vi "ForceSensor_Final.vi"() -> ()   [LabVIEW 2020]
uses:
  <vilib>/Analysis/baseanly.llb/Mean (DBL).vi
  <vilib>/httpClient/PUTBuffer.vi
  <vilib>/httpClient/LabVIEWHTTPClient.lvlib
  <vilib>/ptbypt/NI_PtbyPt.lvlib
  <vilib>/Analysis/NI_AALBase.lvlib
panel:
  out "Waveform Chart 2":dynamicdata(graph)
  out "Cloud payload":string
  out "Waveform Chart":dynamicdata(graph)
  out "x > y?":bool
  in  "Calibration Tap":bool
  in  "Calibration Reset":bool
  out "BPM":dbl
  in  "stop":bool
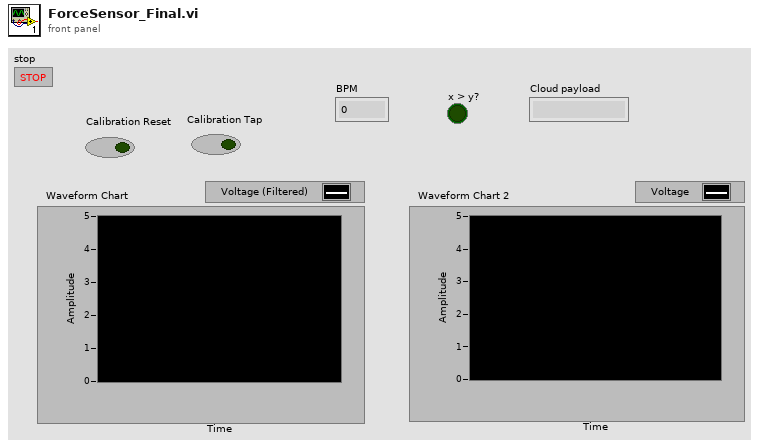
[diagram p1: front panel]
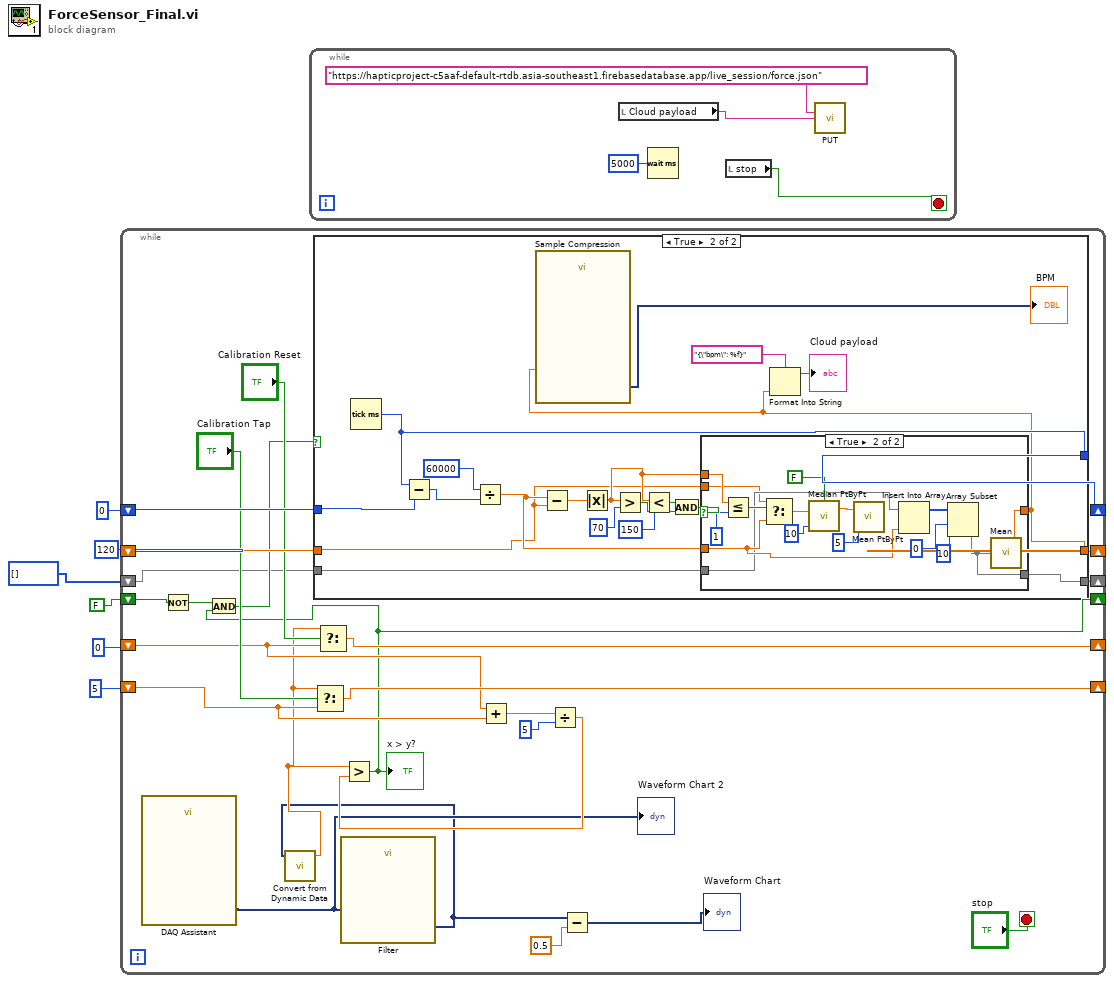
[diagram p0: block diagram]
diagram:
  n1 = while {
    shift-right: [w29] -> _
    shift-left: 0 -> [w30]
    shift-right: [w27] -> _
    shift-left: 120 -> [w28]
    shift-right: [w24] -> _
    shift-left: 0 -> [w22]
    shift-right: [w23] -> _
    shift-left: 5 -> [w21]
    shift-right: [w13] -> _
    shift-left: FALSE -> [w16]
    shift-right: [w11] -> _
    shift-left: i32[] [] -> [w12]
    stop <- "stop" stop-if-true
    n2 = call "DAQ Assistant"() -> ("data"=w10:dynamicdata)  [unwired: 16 in, 3 out]
    "Waveform Chart 2" <- w10
    n3 = Not(x=w16) -> (.not. x?=w15:bool)
    n4 = call "Filter"("Signal"=w10) -> ("Filtered Signal"=w9:dynamicdata)  [unwired: 9 in, 1 out]
    n5 = call "Convert from Dynamic Data"("Dynamic Data Type"=w9) -> ("Scalar"=w17:dbl)  [unwired: 3 in]
    n6 = Select(t=w17, s="Calibration Tap", f=w21) -> (s? t:f=w23:dbl)
    n7 = Select(t=w17, s="Calibration Reset", f=w22) -> (s? t:f=w24:dbl)
    n8 = Add(x=w22, y=w21) -> (x+y=w20:dbl)
    n9 = Divide(x=w20, y=5) -> (x/y=w18:dbl)
    n10 = Greater?(x=w17, y=w18) -> (0:w13:bool)
    "x > y?" <- w13
    n11 = And(x=w15, y=w13) -> (x .and. y?=w14:bool)
    n12 = case shown="True" w14 {
      tunnel: w30 -> [w34 w53]
      tunnel: [w34 w50] -> w29
      tunnel: w28 -> [w33 w37]
      tunnel: [w33 w35] -> w27
      tunnel: w12 -> [w32 w39]
      tunnel: [w32 w38] -> w11
      frame False {
      }
      frame True {
        n13 = Tick Count (ms)() -> (millisecond timer value=w50:u32)
        n14 = Subtract(x=w50, y=w53) -> (x-y=w51:u32)
        n15 = Divide(x=60000, y=w51) -> (x/y=w48:dbl)
        n16 = Subtract(x=w48, y=w37) -> (x-y=w49:dbl)
        n17 = Absolute Value(x=w49) -> (abs(x)=w42:dbl)
        n18 = Greater?(x=w42, y=70) -> (0:w44:bool)
        n19 = Less?(x=w42, y=150) -> (x < y?=w45:bool)
        n20 = And(x=w45, y=w44) -> (x .and. y?=w43:bool)
        n21 = case shown="True" w43 {
          tunnel: [w55 w60] -> w35
          tunnel: w37 -> [_ w56]
          tunnel: w48 -> [w55 w59]
          tunnel: w42 -> [_ w64]
          tunnel: w39 -> [w54 w58]
          tunnel: [w54 w57] -> w38
          frame False {
          }
          frame True {
            n22 = Less Or Equal?(x=w64, y=1) -> (x <= y?=w71:bool)
            n23 = Select(t=w56, s=w71, f=w59) -> (s? t:f=w69:dbl)
            n24 = call <vilib>:"Median PtByPt.vi"("initialize"=FALSE, "sample length"=10, "x"=w69) -> ("median"=w66:dbl)  [unwired: 1 in, 1 out]
            n25 = call <vilib>:"Mean PtByPt.vi"("x"=w66, "sample length"=5) -> ()  [unwired: 2 in, 2 out]
            n26 = Insert Into Array(array=w58, new element=w59) -> (w63:i32[])  [unwired: 1 in]
            n27 = Array Subset(array=w63, index=0, length=10) -> (w57:i32[])
            n28 = call-poly <vilib>:"Mean.vi"("X"=w57) -> ("mean"=w60:dbl)  [unwired: 1 out]
          }
        }
        n29 = call "Sample Compression"("Signals"=w35) -> ("Mean"=→"BPM":dynamicdata)  [unwired: 8 in, 2 out]
        n30 = Format Into String(format string="{\"bpm\": %f}", w35) -> (resulting string=→"Cloud payload":string)  [unwired: 2 in, 1 out]
      }
    }
    n31 = Subtract(x=w9, y=0.5) -> (x-y=→"Waveform Chart":dynamicdata)
  }
  n32 = while {
    stop <- w72 stop-if-true
    n33 = local read "Cloud payload"() -> (w74:string)
    n34 = Wait (ms)(milliseconds to wait=u32 5000) -> ()  [unwired: 1 out]
    n35 = local read "stop"() -> (w72:bool)
    n36 = call-poly <vilib>:"PUT.vi"("url"="https://hapticproject-c5aaf-default-rtdb.asia-southeast1.firebasedatabase.app/live_session/force.json", "buffer"=w74) -> ()  [unwired: 10 in, 4 out]
  }
